vi "Qudi_FTL_QPD_PID.vi"(3 "N Z positions":i32) -> ()   [LabVIEW 2015]
uses:
  <vilib>/rvi/Analysis/control/PID/Typedef/niFpgaPID_PIGains.ctl
  <vilib>/Platform/TimedLoop/XDataNode/timing_clust.ctl
  <vilib>/Platform/TimedLoop/XDataNode/nitl_modes.ctl
  <vilib>/Platform/TimedLoop/XDataNode/wakeup.ctl
  <vilib>/rvi/FXPMathLib/basic elements/FxpIntAccumulator/subVIs/nifxpmath_IntAccumulator_SimConfig.ctl
  <vilib>/rvi/Emulation/niFpgaGetClockAttributes.vi
  <vilib>/rvi/Emulation/niFpgaSctlEmulationGetInTimedLoop.vi
  <vilib>/rvi/Emulation/niFpgaEmulationReportErrorSimple.vi
  <vilib>/rvi/eio/common/nirviEmuTemplateMethod_errors.vi
  <vilib>/rvi/Emulation/niFpgaProcessEmulError.vi
  <vilib>/rvi/Analysis/common/codeGenErrors/XNode/niFpgaXNodeCodeGenErrorHandle.vi
  <vilib>/rvi/Emulation/niFpgaCriticalErrorInLSC.vi
  <vilib>/rvi/FXPMathLib/basic elements/FxpIntAccumulator/simVIs/DllFxpIntAccumulator_sub.vi
  <vilib>/rvi/Analysis/control/PID/SubVIs/niFpgaPID_PIWrapper.vi
  <vilib>/eio/EIONode/EIONode.xnode
  <vilib>/rvi/Analysis/measure/dc-rms/XNode/niFpgaDC-RMS.xnode
  <vilib>/Platform/TimedLoop/XDataNode/XDataNode.xnode
  <vilib>/rvi/FXPMathLib/basic elements/FxpIntAccumulator/XNode/nifxpmath_IntAccumulator.xnode
  <vilib>/rvi/FXPMathLib/FxpMul/XNode/nifxpmath_Multiplier.xnode
  <vilib>/Platform/TimedLoop/XDataNode/XDNodeRunTimeDep.lvlib
  <vilib>/rvi/FXPMathLib/sim/FxpSim.dll
panel:
  in  "exposure_time_ms":u16
  in  "integration_time_us":u32=100 caption="Count(uSec)"
  in  "stop":bool
  out "duration_ms":u32
  out "X":i16
  out "Y":i16
  out "Sum":i16
  out "counter":u32
  out "output":i16
  in  "reset":bool
  in  "reset_counter":bool
  in  "autofocus":bool
  in  "setpoint":i16
  in  "P":i16
  in  "I":i16
  in  "ref_axis":bool
  out "n cycles":i32
  out "Images acquired":i32
  in  "Laser lines":i8[](array[numeric])=[0, 0, 0, 0, 0]
  in  "Laser power":i16[](array[numeric])=[0, 0, 0, 0, 0]
  in  "N laser lines":i32
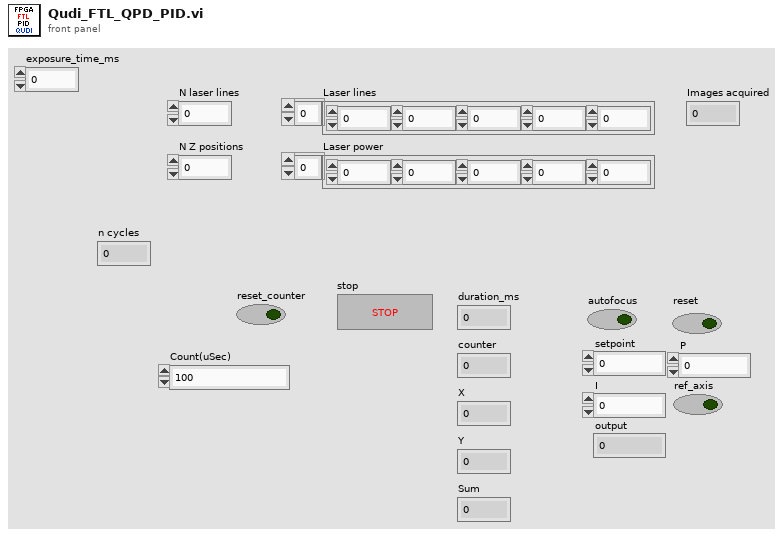
[diagram p1: front panel]
types:
  T1 = typedef "niFpgaPID_PIGains.ctl" = cluster{"proportional gain":sgl, "integral gain":sgl}
  T2 = typedef "XDNodeRunTimeDep.lvlib/timing_clust.ctl" = cluster{"Expected End [f-1]":u64, "Actual End [f-1]":u64, "Finished Late? [f-1]":bool, "Expected End [i-1]":u64, "Actual End [i-1]":u64, "Finished Late? [i-1]":bool, "Expected Start [i]":u64, "Actual Start [i]":u64, "Expected Start [f]":u64, "Actual Start [f]":u64, "Source Name":string, "Structure Name":string, "Period":i64, "Deadline":i64, "Offset":i64, "Start":i64, "Priority":i32, "Timeout":i32, "Mode":T3, "Wakeup Reason":T4, "Error":errorcluster, "Source Type":string, "Secondary Source Type":string, "Global End Time":u64, "Global Start Time":u64, "Frame Duration":u64, "Iteration Duration":u64, "Assigned CPU":i32, "I/O Scan Engine Mode":u32}
  T3 = typedef "XDNodeRunTimeDep.lvlib/nitl_modes.ctl" = enum32{"No Change", "Process missed periods, maintain original phase", "Discard missed periods, maintain original phase", "Process missed periods, ignore original phase", "Discard missed periods, ignore original phase"}
  T4 = typedef "XDNodeRunTimeDep.lvlib/wakeup.ctl" = enum32{"Normal", "Aborted", "Asynchronous wakeup", "Timing source error", "Timed loop error", "Timeout"}
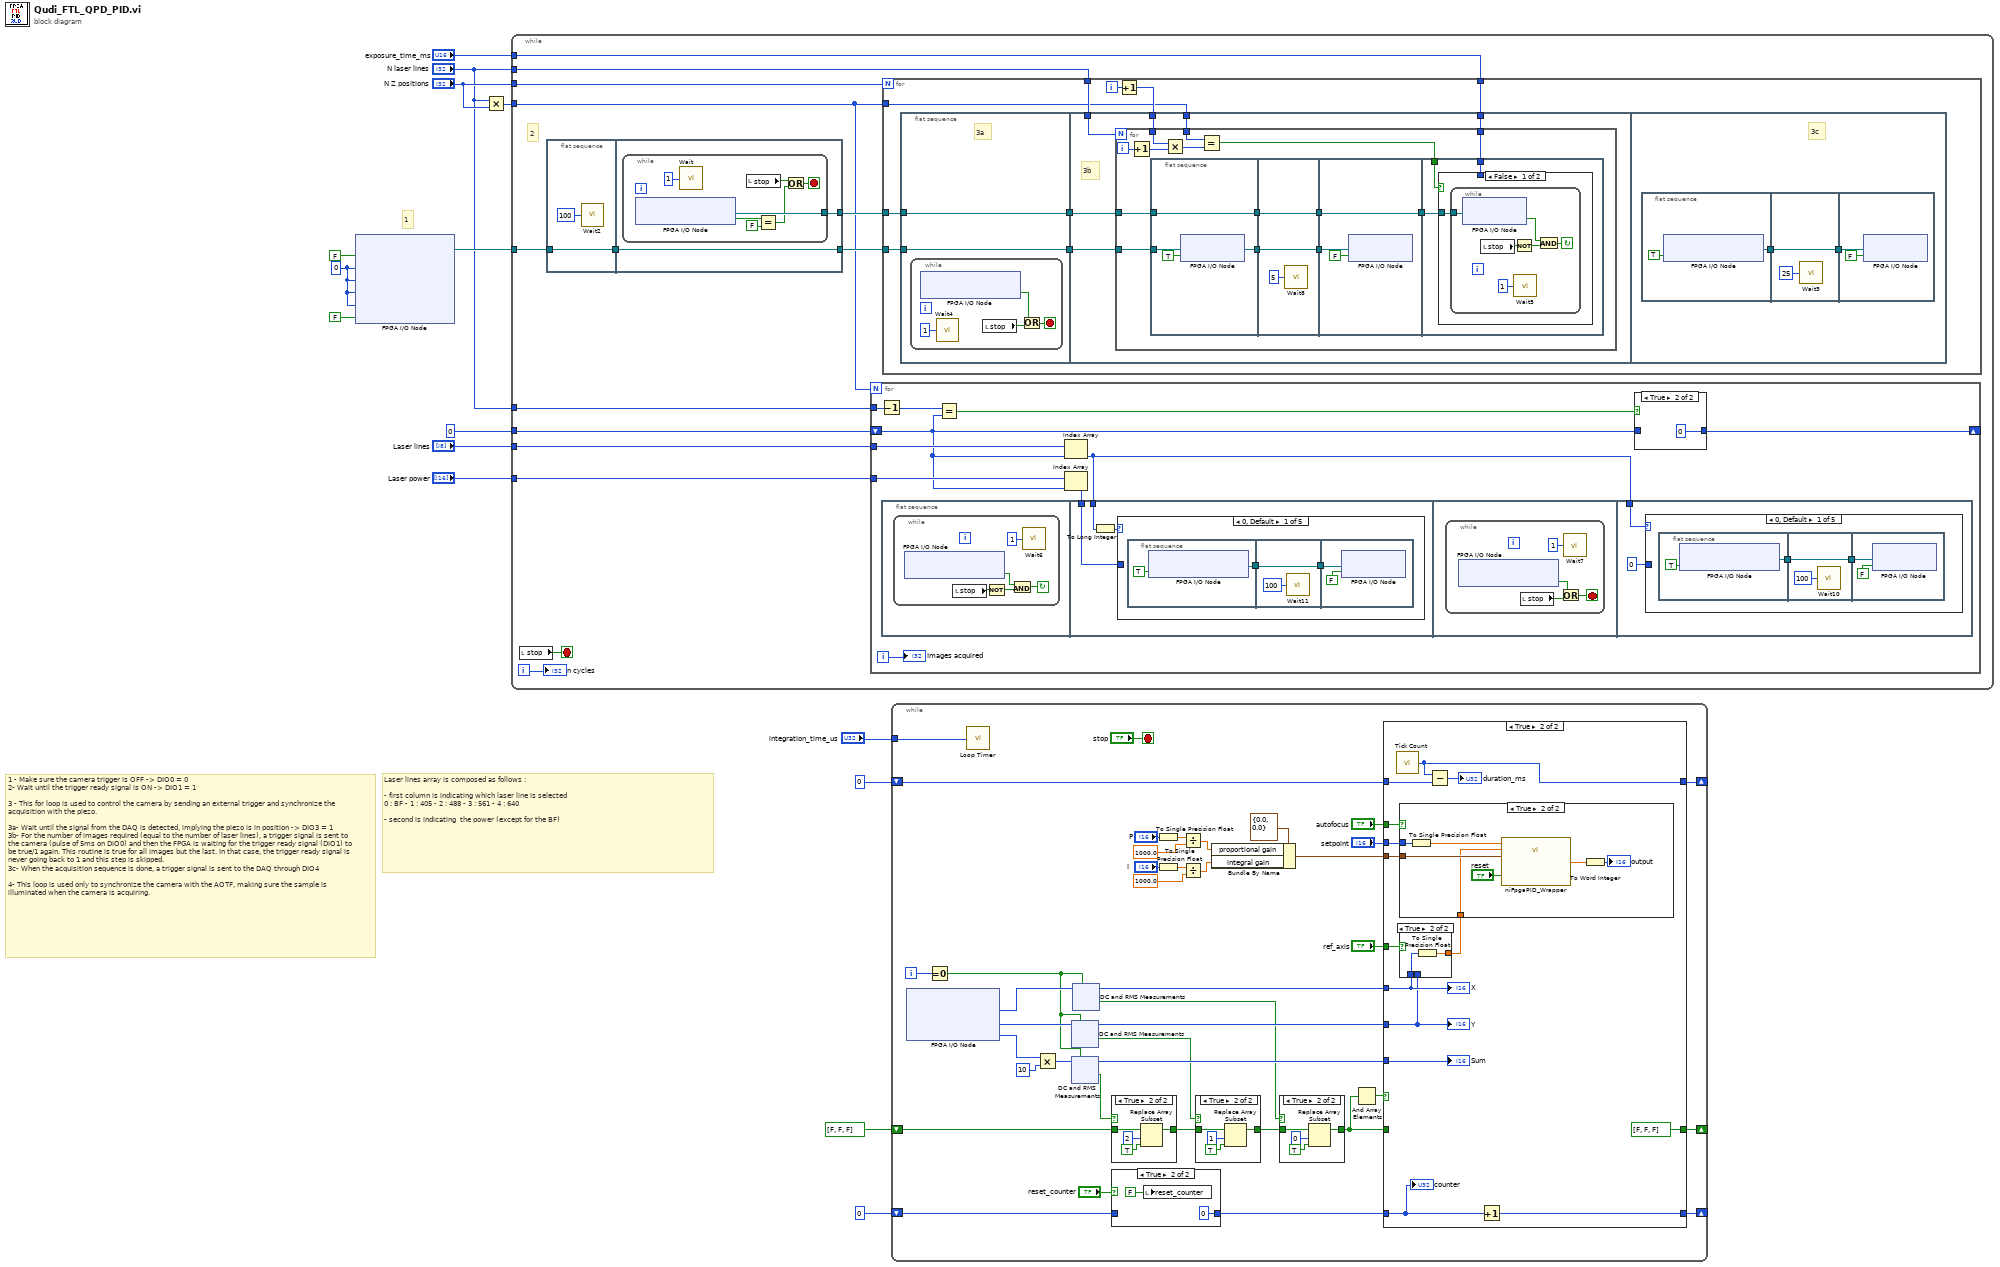
[diagram p0: block diagram]
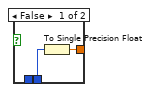
[diagram p7: hidden frame]
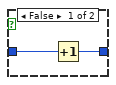
[diagram p9: hidden frame]
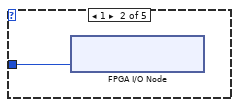
[diagram p10: hidden frame]
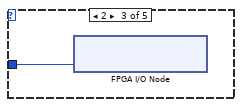
[diagram p11: hidden frame]
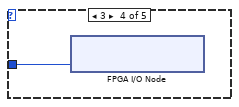
[diagram p12: hidden frame]
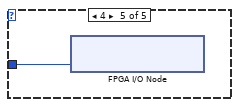
[diagram p13: hidden frame]
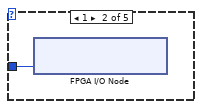
[diagram p14: hidden frame]
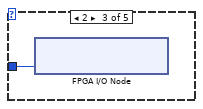
[diagram p15: hidden frame]
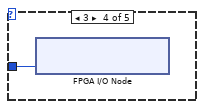
[diagram p16: hidden frame]
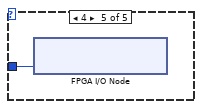
[diagram p17: hidden frame]
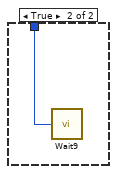
[diagram p18: hidden frame]
diagram:
  w10 = i16 0 ("Connector0/AO0")
  # "Laser lines array is composed as follows :\n\n- first column is indicating which laser line is selected \n0 : BF - 1 : 405 - 2 : 488 - 3 : 561 - 4 : 640\n\n- second is indicating  the power (except for the BF)"
  # "1"
  # "1 - Make sure the camera trigger is OFF -> DIO0 = 0\n2- Wait until the trigger ready signal is ON -> DIO1 = 1\n\n3 - This for loop is used to control the camera by sending an external trigger and synchronize the acquisition with the piezo.\n\n3a- Wait until the signal from the DAQ is detected, implying the piezo is in position -> DIO3 = 1 \n3b- For the number of images required (equal to the number of laser lines), a trigger signal is sent to the camera (pulse of 5ms on DIO0) and then the FPGA is waiting for the trigger ready signal (DIO1) to be true/1 again. This routine is true for all images but the last. In that case, the trigger ready signal is never going back to 1 and this step is skipped. \n3c- When the acquisition sequence is done, a trigger signal is sent to the DAQ through DIO4\n\n4- This loop is used only to synchronize the camera with the AOTF, making sure the sample is illuminated when the camera is acquiring."
  n1 = xnode "FPGA I/O Node"("Connector0/DIO0"=FALSE, "Connector0/AO0"=w10, "Connector0/AO1"=w10, "Connector0/AO2"=w10, "Connector0/AO3"=w10, "Connector0/DIO5"=FALSE) -> ("FPGA I/O Out"=w14:refnum<k21>)  [unwired: 6 in, 5 out]
  n2 = Multiply(x="N laser lines", y="N Z positions") -> (x*y=w3:i32)
  n3 = while {
    tunnel: w14 -> [w28]
    tunnel: "Laser power" -> [w25]
    tunnel: "Laser lines" -> [w24]
    tunnel: 0 -> [w23]
    tunnel: "N Z positions" -> [w22]
    tunnel: "N laser lines" -> [w19]
    tunnel: w3 -> [w18]
    tunnel: "N laser lines" -> [w17]
    tunnel: "exposure_time_ms" -> [w16]
    i -> [w20]
    stop <- w21 stop-if-true
    # "2"
    n4 = local read "stop"() -> (w21:bool)
    n5 = flat-sequence {
      tunnel: w28 -> [w82]
      tunnel: [w82] -> w29
      tunnel: w29 -> [w84]
      tunnel: [w84] -> w27
      tunnel: [w83] -> w26
      frame #0 {
        n6 = call "Wait2"("Count(uSec)"=u8 100 ("Count(mSec)")) -> ()  [unwired: 1 out]
      }
      frame #1 {
        n7 = while {
          tunnel: [w91] -> w83
          stop <- w86 stop-if-true
          n8 = xnode "FPGA I/O Node"() -> ("Connector0/DIO1"=w90:bool, "FPGA I/O Out"=w91:refnum<k21>)  [unwired: 1 in]
          n9 = call "Wait"("Count(mSec)"=u8 1) -> ()  [unwired: 1 out]
          n10 = local read "stop"() -> (w87:bool)
          n11 = Equal?(x=w90, y=FALSE) -> (x = y?=w88:bool)
          n12 = Or(x=w87, y=w88) -> (x .or. y?=w86:bool)
        }
      }
    }
    n13 = for {
      N: w18 -> [_]
      shift-right: [w37] -> _
      shift-left: w23 -> [w34]
      tunnel: w24 -> [w36]
      tunnel: w25 -> [w35]
      tunnel: w17 -> [w32]
      i -> [w30]
      n14 = Decrement(x=w32) -> (x-1=w31:i32)
      n15 = flat-sequence {
        tunnel: w39 -> [w49]
        tunnel: w33 -> [w48]
        tunnel: w39 -> [w67]
        frame #0 {
          n16 = while {
            stop <- w44 continue-if-true
            n17 = xnode "FPGA I/O Node"() -> ("Connector0/DIO2"=w45:bool)  [unwired: 1 in, 1 out]
            n18 = local read "stop"() -> (w46:bool)
            n19 = Not(x=w46) -> (.not. x?=w47:bool)
            n20 = And(x=w45, y=w47) -> (x .and. y?=w44:bool)
            n21 = call "Wait6"("Count(mSec)"=u8 1) -> ()  [unwired: 1 out]
          }
        }
        frame #1 {
          n22 = To Long Integer(number=w49) -> (32bit integer=w50:i32)
          n23 = case shown="0, Default" w50 {
            tunnel: w48 -> [_ w59 w60 w61 w62]
            frame 0, Default {
              n24 = flat-sequence {
                tunnel: [w53] -> w52
                tunnel: w52 -> [w55]
                tunnel: [w55] -> w51
                tunnel: w51 -> [w58]
                frame #0 {
                  n25 = xnode "FPGA I/O Node"("Connector0/DIO5"=TRUE) -> ("FPGA I/O Out"=w53:refnum<k21>)  [unwired: 1 in]
                }
                frame #1 {
                  n26 = call "Wait11"("Count(uSec)"=u32 100) -> ()  [unwired: 1 out]
                }
                frame #2 {
                  n27 = xnode "FPGA I/O Node"("I/O Item"=FALSE, "FPGA I/O In"=w58) -> ()  [unwired: 1 out]
                }
              }
            }
            frame 1 {
              n28 = xnode "FPGA I/O Node"("Connector0/AO2"=w59) -> ()  [unwired: 1 in, 1 out]
            }
            frame 2 {
              n29 = xnode "FPGA I/O Node"("Connector0/AO3"=w60) -> ()  [unwired: 1 in, 1 out]
            }
            frame 3 {
              n30 = xnode "FPGA I/O Node"("Connector0/AO0"=w61) -> ()  [unwired: 1 in, 1 out]
            }
            frame 4 {
              n31 = xnode "FPGA I/O Node"("Connector0/AO1"=w62) -> ()  [unwired: 1 in, 1 out]
            }
          }
        }
        frame #2 {
          n32 = while {
            stop <- w64 stop-if-true
            n33 = xnode "FPGA I/O Node"() -> ("Connector0/DIO2"=w65:bool)  [unwired: 1 in, 1 out]
            n34 = local read "stop"() -> (w66:bool)
            n35 = Or(x=w65, y=w66) -> (x .or. y?=w64:bool)
            n36 = call "Wait7"("Count(mSec)"=u8 1) -> ()  [unwired: 1 out]
          }
        }
        frame #3 {
          n37 = case shown="0, Default" w67 {
            tunnel: i16 0 -> [_ w77 w78 w79 w80]
            frame 0, Default {
              n38 = flat-sequence {
                tunnel: [w71] -> w70
                tunnel: w70 -> [w73]
                tunnel: [w73] -> w69
                tunnel: w69 -> [w76]
                frame #0 {
                  n39 = xnode "FPGA I/O Node"("Connector0/DIO5"=TRUE) -> ("FPGA I/O Out"=w71:refnum<k21>)  [unwired: 1 in]
                }
                frame #1 {
                  n40 = call "Wait10"("Count(uSec)"=u32 100) -> ()  [unwired: 1 out]
                }
                frame #2 {
                  n41 = xnode "FPGA I/O Node"("I/O Item"=FALSE, "FPGA I/O In"=w76) -> ()  [unwired: 1 out]
                }
              }
            }
            frame 1 {
              n42 = xnode "FPGA I/O Node"("Connector0/AO2"=w77) -> ()  [unwired: 1 in, 1 out]
            }
            frame 2 {
              n43 = xnode "FPGA I/O Node"("Connector0/AO3"=w78) -> ()  [unwired: 1 in, 1 out]
            }
            frame 3 {
              n44 = xnode "FPGA I/O Node"("Connector0/AO0"=w79) -> ()  [unwired: 1 in, 1 out]
            }
            frame 4 {
              n45 = xnode "FPGA I/O Node"("Connector0/AO1"=w80) -> ()  [unwired: 1 in, 1 out]
            }
          }
        }
      }
      n46 = Equal?(x=w31, y=w34) -> (x = y?=w38:bool)
      n47 = Index Array(array=w36, index=w34) -> (element=w39:i8)
      n48 = Index Array(array=w35, index=w34) -> (element=w33:i16)
      n49 = case shown="True" w38 {
        tunnel: w34 -> [w41 _]
        tunnel: [w40 0] -> w37
        frame False {
          n50 = Increment(x=w41) -> (x+1=w40:i32)
        }
        frame True {
        }
      }
      "Images acquired" <- w30
    }
    n51 = for {
      N: w22 -> [_]
      tunnel: w27 -> [w99]
      tunnel: w26 -> [w100]
      tunnel: w19 -> [w95]
      tunnel: w18 -> [w93]
      tunnel: w16 -> [w92]
      i -> [w96]
      n52 = flat-sequence {
        tunnel: w99 -> [w101]
        tunnel: w100 -> [w102]
        tunnel: [w102] -> w98
        tunnel: [w101] -> w97
        tunnel: w98 -> [w112]
        tunnel: w97 -> [w111]
        tunnel: w95 -> [w110]
        tunnel: w94 -> [w109]
        tunnel: w93 -> [w108]
        tunnel: w92 -> [w107]
        frame #0 {
          # "3a"
          n53 = while {
            stop <- w104 stop-if-true
            n54 = xnode "FPGA I/O Node"() -> ("Connector0/DIO3"=w105:bool)  [unwired: 1 in, 1 out]
            n55 = call "Wait4"("Count(mSec)"=u8 1) -> ()  [unwired: 1 out]
            n56 = local read "stop"() -> (w106:bool)
            n57 = Or(x=w105, y=w106) -> (x .or. y?=w104:bool)
          }
        }
        frame #1 {
          # "3b"
          n58 = for {
            N: w110 -> [_]
            tunnel: w112 -> [w121]
            tunnel: w111 -> [w120]
            tunnel: w109 -> [w117]
            tunnel: w108 -> [w115]
            tunnel: w107 -> [w113]
            i -> [w119]
            n59 = Increment(x=w119) -> (x+1=w118:i32)
            n60 = flat-sequence {
              tunnel: [w129] -> w126
              tunnel: [w127] -> w125
              tunnel: w120 -> [w128]
              tunnel: w121 -> [w127]
              tunnel: w126 -> [w133]
              tunnel: [w133] -> w124
              tunnel: [w132] -> w123
              tunnel: w125 -> [w132]
              tunnel: w124 -> [w135]
              tunnel: [w134] -> w122
              tunnel: w123 -> [w134]
              tunnel: w122 -> [w139]
              tunnel: w114 -> [w138]
              tunnel: w113 -> [w137]
              frame #0 {
                n61 = xnode "FPGA I/O Node"("I/O Item"=TRUE ("Connector0/DIO0"), "FPGA I/O In"=w128) -> ("FPGA I/O Out"=w129:refnum<k21>)
              }
              frame #1 {
                n62 = call "Wait8"("Count(mSec)"=u8 5) -> ()  [unwired: 1 out]
              }
              frame #2 {
                n63 = xnode "FPGA I/O Node"("I/O Item"=FALSE ("Connector0/DIO0"), "FPGA I/O In"=w135) -> ()  [unwired: 1 out]
              }
              frame #3 {
                n64 = case shown="False" w138 {
                  tunnel: w139 -> [w140 _]
                  tunnel: w137 -> [_ w147]
                  frame False {
                    n65 = while {
                      tunnel: w140 -> [w146]
                      stop <- w142 continue-if-true
                      n66 = xnode "FPGA I/O Node"("FPGA I/O In"=w146) -> ("I/O Item"=w143:bool)  [unwired: 1 out]
                      n67 = local read "stop"() -> (w145:bool)
                      n68 = Not(x=w145) -> (.not. x?=w144:bool)
                      n69 = call "Wait5"("Count(mSec)"=u8 1) -> ()  [unwired: 1 out]
                      n70 = And(x=w143, y=w144) -> (x .and. y?=w142:bool)
                    }
                  }
                  frame True {
                    n71 = call "Wait9"("Count(mSec)"=w147) -> ()  [unwired: 1 out]
                  }
                }
              }
            }
            n72 = Multiply(x=w117, y=w118) -> (x*y=w116:i32)
            n73 = Equal?(x=w115, y=w116) -> (x = y?=w114:bool)
          }
        }
        frame #2 {
          # "3c"
          n74 = flat-sequence {
            tunnel: [w151] -> w149
            tunnel: w149 -> [w152]
            tunnel: [w152] -> w148
            tunnel: w148 -> [w154]
            frame #0 {
              n75 = xnode "FPGA I/O Node"("Connector0/DIO4"=TRUE) -> ("FPGA I/O Out"=w151:refnum<k21>)  [unwired: 1 in]
            }
            frame #1 {
              n76 = call "Wait3"("Count(mSec)"=u8 25) -> ()  [unwired: 1 out]
            }
            frame #2 {
              n77 = xnode "FPGA I/O Node"("I/O Item"=FALSE ("Connector0/DIO0"), "FPGA I/O In"=w154) -> ()  [unwired: 1 out]
            }
          }
        }
      }
      n78 = Increment(x=w96) -> (x+1=w94:i32)
    }
    "n cycles" <- w20
  }
  n79 = while {
    shift-right: [w179] -> _
    shift-left: bool[] [FALSE, FALSE, FALSE] ("initialized array") -> [w187]
    shift-right: [w177] -> _
    shift-left: u32 0 -> [w178]
    tunnel: "integration_time_us" -> [w176]
    shift-right: [w175] -> _
    shift-left: u32 0 -> [w173]
    i -> [w193]
    stop <- "stop" stop-if-true
    n80 = xnode "FPGA I/O Node"() -> ("Connector0/AI0"=w195:i16, "Connector0/AI1"=w191:i16, "Connector0/AI2"=w158:i16)  [unwired: 3 in, 3 out]
    n81 = Equal To 0?(x=w193) -> (x = 0?=w188:bool)
    n82 = call "Loop Timer"("Count(uSec)"=w176) -> ()  [unwired: 1 out]
    n83 = Multiply(x=w158, y=i16 10) -> (x*y=w157:i16)
    n84 = xnode "DC and RMS Measurements"("input data"=w191, "reset"=w188) -> ("DC"=w190:i16, "output valid"=w183:bool)
    n85 = xnode "DC and RMS Measurements"("input data"=w157, "reset"=w188) -> ("DC"=w189:i16, "output valid"=w184:bool)
    n86 = xnode "DC and RMS Measurements"("input data"=w195, "reset"=w188) -> ("DC"=w192:i16, "output valid"=w182:bool)
    n87 = case shown="True" w184 {
      tunnel: w187 -> [w204 w207]
      tunnel: [w204 w205] -> w186
      frame False {
      }
      frame True {
        n88 = Replace Array Subset(array=w207, new element=TRUE, index=2) -> (w205:bool[])
      }
    }
    n89 = case shown="True" "reset_counter" {
      tunnel: w173 -> [w196 _]
      tunnel: [w196 u32 0] -> w172
      frame False {
      }
      frame True {
        n90 = local write "reset_counter"(FALSE ("Reset counter")) -> ()
      }
    }
    n91 = To Single Precision Float(number="P") -> (single precision float=w165:sgl)
    n92 = To Single Precision Float(number="I") -> (single precision float=w162:sgl)
    n93 = Divide(x=w165, y=sgl 1000.0) -> (x/y=w163:sgl)
    n94 = Divide(x=w162, y=sgl 1000.0) -> (x/y=w160:sgl)
    n95 = case shown="True" w183 {
      tunnel: w186 -> [w209 w212]
      tunnel: [w209 w210] -> w185
      frame False {
      }
      frame True {
        n96 = Replace Array Subset(array=w212, new element=TRUE, index=1) -> (w210:bool[])
      }
    }
    n97 = Bundle By Name(cluster=T1 {"proportional gain"=0.0, "integral gain"=0.0} ("gains"), "proportional gain"=w163, "integral gain"=w160) -> (w166:T1)
    n98 = case shown="True" w182 {
      tunnel: [w199 w201] -> w180
      tunnel: w185 -> [w199 w200]
      frame False {
      }
      frame True {
        n99 = Replace Array Subset(array=w200, new element=TRUE, index=0) -> (w201:bool[])
      }
    }
    n100 = And Array Elements(Boolean array=w180) -> (logical AND=w181:bool)
    n101 = case shown="True" w181 {
      tunnel: w192 -> [_ w219]
      tunnel: w190 -> [_ w217]
      tunnel: w189 -> [_ w225]
      tunnel: w180 -> [w216 _]
      tunnel: [w216 bool[] [FALSE, FALSE, FALSE] ("initialized array")] -> w179
      tunnel: w178 -> [w215 w229]
      tunnel: [w215 w227] -> w177
      tunnel: w172 -> [w214 w224]
      tunnel: [w214 w226] -> w175
      tunnel: "autofocus" -> [_ w223]
      tunnel: "setpoint" -> [_ w222]
      tunnel: w166 -> [_ w221]
      tunnel: "ref_axis" -> [_ w220]
      frame False {
      }
      frame True {
        n102 = call "Tick Count"() -> ("Tick Count(mSec)"=w227:u32)
        n103 = case shown="True" w220 {
          tunnel: w219 -> [_ w234]
          tunnel: [w231 w233] -> w218
          tunnel: w217 -> [w232 _]
          frame False {
            n104 = To Single Precision Float(number=w232) -> (single precision float=w231:sgl)
          }
          frame True {
            n105 = To Single Precision Float(number=w234) -> (single precision float=w233:sgl)
          }
        }
        n106 = case shown="True" w223 {
          tunnel: w222 -> [_ w241]
          tunnel: w221 -> [_ w239]
          tunnel: w218 -> [_ w235]
          frame False {
          }
          frame True {
            n107 = To Single Precision Float(number=w241) -> (single precision float=w240:sgl)
            n108 = call-poly <vilib>:"niFpgaPID_Wrapper.vi"("setpoint"=w240, "reset? (F)"="reset", "process variable"=w235, "gains"=w239) -> ("output"=w237:sgl)  [unwired: 9 in, 2 out]
            n109 = To Word Integer(number=w237) -> (16bit integer=→"output":i16)
          }
        }
        n110 = Subtract(x=w227, y=w229) -> (x-y=→"duration_ms":u32)
        n111 = Increment(x=w224) -> (x+1=w226:u32)
        "X" <- w219
        "Y" <- w217
        "Sum" <- w225
        "counter" <- w224
      }
    }
  }
